vi "DAQmx Synchronized Control.vi"() -> ()   [LabVIEW 2025]
uses:
  <vilib>/Utility/error.llb/DialogType.ctl
  <vilib>/DAQmx/read.llb/DAQmx Read (Analog 1D DBL NChan 1Samp).vi
  <vilib>/DAQmx/write.llb/DAQmx Write (Analog 1D DBL NChan 1Samp).vi
  <vilib>/DAQmx/create/channels.llb/DAQmx Create Channel (AI-Voltage-Basic).vi
  <vilib>/DAQmx/configure/timing.llb/DAQmx Timing (Sample Clock).vi
  <vilib>/DAQmx/create/channels.llb/DAQmx Create Channel (AO-Voltage-Basic).vi
  <vilib>/DAQmx/miscellaneous.llb/DAQmx Fill In Error Info.vi
  <resource>/objmgr/daqmx.rc
panel:
  in  "Gen Data":dbl
  out "SampClk.Term":tag
  out "Waveform Chart":dbl[][](graph)
  in  "Stop":bool
  in  "Sample Rate":dbl=500.0
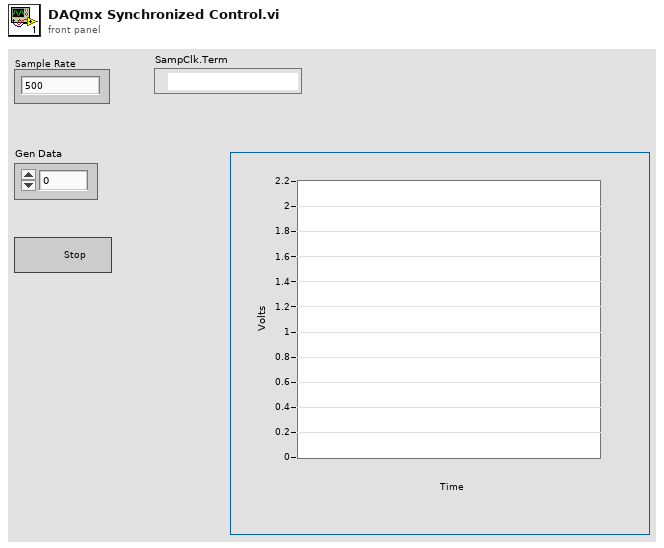
[diagram p1: front panel]
types:
  T1 = typedef "DialogType.ctl" = u16
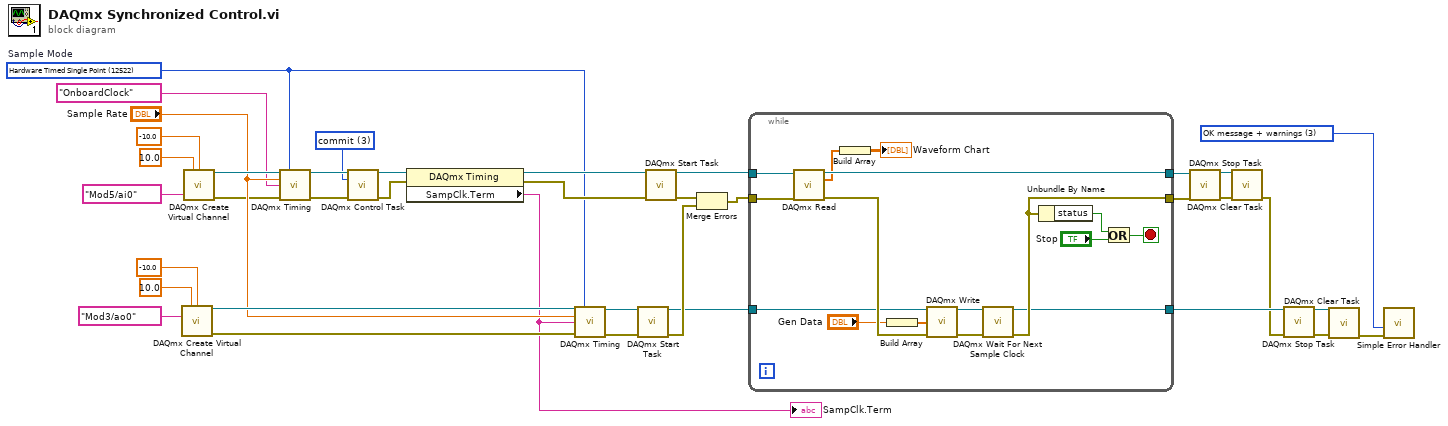
[diagram p0: block diagram]
diagram:
  w8 = 3 items=["verify"=2, "reserve"=4, "commit"=3, "unreserve"=5, "abort"=6] ("action")
  w29 = T1 3 items=["no dialog", "OK message", "continue or stop message", "OK message + warnings", "continue/stop + warnings"] ("type of dialog (OK msg:1)")
  w1 = 12522 items=["Finite Samples"=10178, "Continuous Samples"=10123, "Hardware Timed Single Point"=12522]  # Sample Mode
  n1 = call-poly <vilib>:"DAQmx Create Virtual Channel.vi"("maximum value"=10.0 ("AO Max Voltage"), "minimum value"=-10.0 ("AO Min Voltage"), "physical channels"=tag "Mod3/ao0" ("AO Physical Channel")) -> ("task out"=w28:refnum<k21>, "error out"=w18:errorcluster)  [unwired: 11 in]
  n2 = call-poly <vilib>:"DAQmx Create Virtual Channel.vi"("maximum value"=10.0 ("AI Max Voltage"), "minimum value"=-10.0 ("AI Min Voltage"), "physical channels"=tag "Mod5/ai0" ("AI Physical Channel")) -> ("task out"=w38:refnum<k21>, "error out"=w17:errorcluster)  [unwired: 11 in]
  n3 = call-poly <vilib>:"DAQmx Timing.vi"("task/channels in"=w38, "sample mode"=w1, "rate"="Sample Rate", "source"=tag "OnboardClock", "error in"=w17) -> ("task out"=w12:refnum<k21>, "error out"=w7:errorcluster)  [unwired: 9 in]
  n4 = call <vilib>:"DAQmx Control Task.vi"("task/channels in"=w12, "action"=w8, "error in"=w7) -> ("task out"=w9:refnum<k21>, "error out"=w5:errorcluster)  [unwired: 11 in]
  n5 = property class="DAQmx Timing"(reference=w9, error in=w5) -> (reference out=w6:refnum<k21>, error out=w4:errorcluster, "SampClk.Term"=w2:tag)
  "SampClk.Term" <- w2
  n6 = call-poly <vilib>:"DAQmx Timing.vi"("task/channels in"=w28, "sample mode"=w1, "rate"="Sample Rate", "source"=w2, "error in"=w18) -> ("task out"=w11:refnum<k21>, "error out"=w10:errorcluster)  [unwired: 9 in]
  n7 = call <vilib>:"DAQmx Start Task.vi"("task/channels in"=w11, "error in"=w10) -> ("task out"=w13:refnum<k21>, "error out"=w16:errorcluster)  [unwired: 12 in]
  n8 = call <vilib>:"DAQmx Start Task.vi"("task/channels in"=w6, "error in"=w4) -> ("task out"=w37:refnum<k21>, "error out"=w15:errorcluster)  [unwired: 12 in]
  n9 = Merge Errors(w15, w16) -> (w14:errorcluster)
  n10 = while {
    tunnel: w37 -> [w44]
    tunnel: w14 -> [w43]
    tunnel: [w51] -> w33
    tunnel: [w46] -> w32
    tunnel: [w45] -> w21
    tunnel: w13 -> [w42]
    stop <- w52 stop-if-true
    n11 = call-poly <vilib>:"DAQmx Read.vi"("task/channels in"=w44, "error in"=w43) -> ("task out"=w51:refnum<k21>, "data"=w41:dbl[], "error out"=w47:errorcluster)  [unwired: 11 in]
    n12 = Build Array(w41) -> (→"Waveform Chart":dbl[][])
    n13 = Build Array("Gen Data") -> (w39:dbl[])
    n14 = call-poly <vilib>:"DAQmx Write.vi"("task/channels in"=w42, "data"=w39, "error in"=w47) -> ("task out"=w49:refnum<k21>, "error out"=w48:errorcluster)  [unwired: 10 in, 1 out]
    n15 = call <vilib>:"DAQmx Wait For Next Sample Clock.vi"("task/channels in"=w49, "error in"=w48) -> ("task out"=w45:refnum<k21>, "error out"=w46:errorcluster)  [unwired: 11 in, 1 out]
    n16 = Unbundle By Name(w46) -> ("status"=w53:bool)
    n17 = Or(x=w53, y="Stop") -> (x .or. y?=w52:bool)
  }
  n18 = call <vilib>:"DAQmx Stop Task.vi"("task/channels in"=w33, "error in"=w32) -> ("task out"=w30:refnum<k21>, "error out"=w31:errorcluster)  [unwired: 12 in]
  n19 = call <vilib>:"DAQmx Clear Task.vi"("task in"=w30, "error in"=w31) -> ("error out"=w20:errorcluster)  [unwired: 13 in]
  n20 = call <vilib>:"DAQmx Stop Task.vi"("task/channels in"=w21, "error in"=w20) -> ("task out"=w24:refnum<k21>, "error out"=w23:errorcluster)  [unwired: 12 in]
  n21 = call <vilib>:"DAQmx Clear Task.vi"("task in"=w24, "error in"=w23) -> ("error out"=w19:errorcluster)  [unwired: 13 in]
  n22 = call <vilib>:"Simple Error Handler.vi"("type of dialog (OK msg:1)"=w29, "error in (no error)"=w19) -> ()  [unwired: 3 in, 5 out]
